vi "Scan DQMH Modules and create Maps.vi"(6 "TreeControl in":refnum<vi>, 7 "Data Cluster In":T2, 8 "error in":errorcluster, 11 "Scan DQMH Modules Argument":T1) -> (0 "error out":errorcluster, 5 "Data Cluster Out":T2={"Maps"={"Tree Map"={}}, "DQMH Scan Results"={"All DQMH Modules Refs"=[], "All Modules Descriptions"=[], "All Modules type"=[], "Project References"={"Project Ref"=refnum, "Project Name"="", "Target"=refnum, "App Ref"=refnum}, "Dependencies"=[]}, "Current Selection"={"VI Ref"=refnum, "DQMH Lib Ref"=refnum}, "Module type"=enum."Singleton", "Module ID"=-1, "Theme"=FALSE, "Broadcast?"=FALSE, "Root Path"="", "Tree Selection"=""})   [LabVIEW 2019, in "Panther Dashboard.lvlib"]
doc: "Gets the Singleton and Cloneable references and creates a list of each type of DQMH Modules"
uses:
  Panther Dashboard.lvlib
  Module Data--cluster.ctl
  Maps List and refs--cluster.ctl
  <vilib>/National Instruments/Tree Map/Tree Map Data.ctl
  DQMH Modules Info--cluster.ctl
  Module type--enum.ctl
  Project References--cluster.ctl
  Scan DQMH Modules Argument--cluster.ctl
  <vilib>/National Instruments/Tree Map/API/List Roots.vi
  <vilib>/National Instruments/Tree Map/Utility/Into Tree Control Items.vi
  <vilib>/Delacor/Delacor QMH/Libraries/Scripting API/DQMH_Scripting API.lvlib
  <vilib>/National Instruments/Tree Map/Tree Map.lvlib
panel:
  out "Pretty XML":string
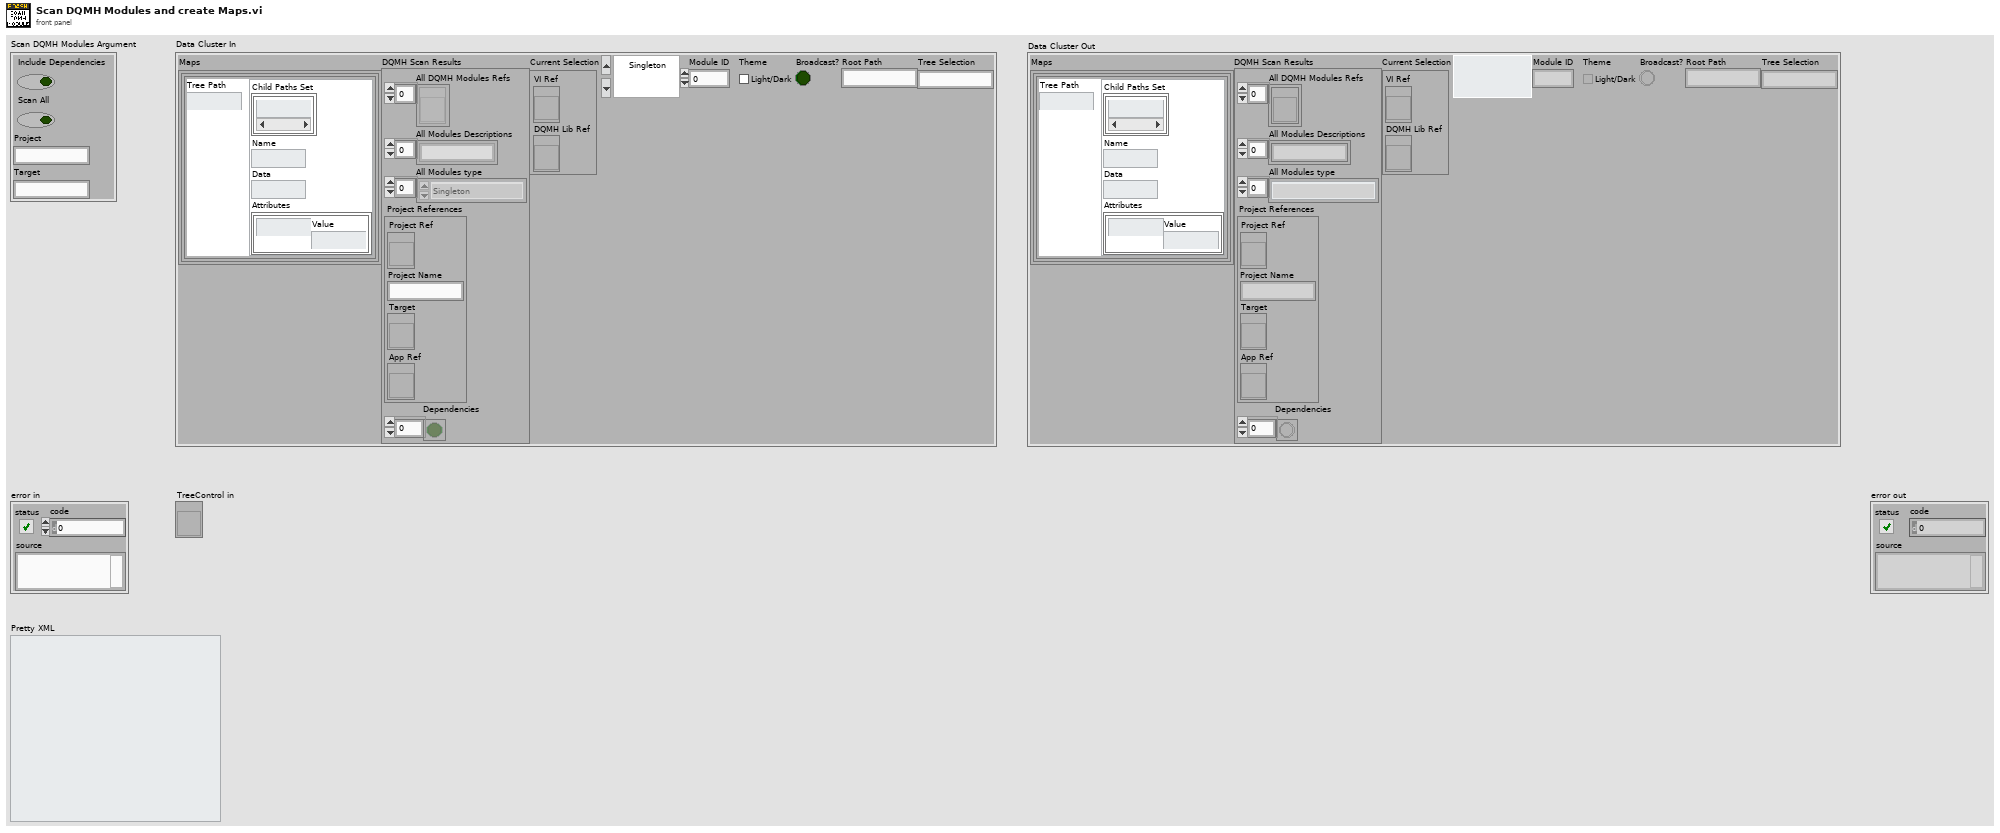
[diagram p1: front panel]
types:
  T1 = typedef "Panther Dashboard.lvlib/Scan DQMH Modules Argument--cluster.ctl" = cluster{"Include Dependencies":bool, "Scan All":bool, "Project":string, "Target":string}
  T2 = typedef "Panther Dashboard.lvlib/Module Data--cluster.ctl" = cluster{"Maps":T3, "DQMH Scan Results":T5, "Current Selection":cluster{"VI Ref":refnum<vi>, "DQMH Lib Ref":refnum<vi>}, "Module type":T6, "Module ID":i32, "Theme":bool, "Broadcast?":bool, "Root Path":string, "Tree Selection":string}
  T3 = typedef "Panther Dashboard.lvlib/Maps List and refs--cluster.ctl" = cluster{"Tree Map":T4}
  T4 = typedef "Tree Map.lvlib/Tree Map Data.ctl" = map{string, cluster{"Child Paths Set":set{string}, "Name":string, "Data":string, "Attributes":map{string, string}}}
  T5 = typedef "Panther Dashboard.lvlib/DQMH Modules Info--cluster.ctl" = cluster{"All DQMH Modules Refs":refnum<vi>[], "All Modules Descriptions":string[], "All Modules type":T6[], "Project References":T7, "Dependencies":bool[]}
  T6 = typedef "Panther Dashboard.lvlib/Module type--enum.ctl" = enum16{"Singleton", "Cloneable"}
  T7 = typedef "Panther Dashboard.lvlib/Project References--cluster.ctl" = cluster{"Project Ref":refnum<vi>, "Project Name":string, "Target":refnum<vi>, "App Ref":refnum<vi>}
  T8 = typedef "DQMH_Scripting API.lvlib/Module Information--cluster.ctl" = cluster{"Library":refnum<vi>, "Qualified Name":string, "Path":path, "Cloneable":bool, "Under Dependencies":bool}
  T9 = cluster{"Left Cell String":string, "Child Text":string[], "Child Tag":string, "Item Indent":i32, "Child Only?":bool, "Glyph Index":i32}[]
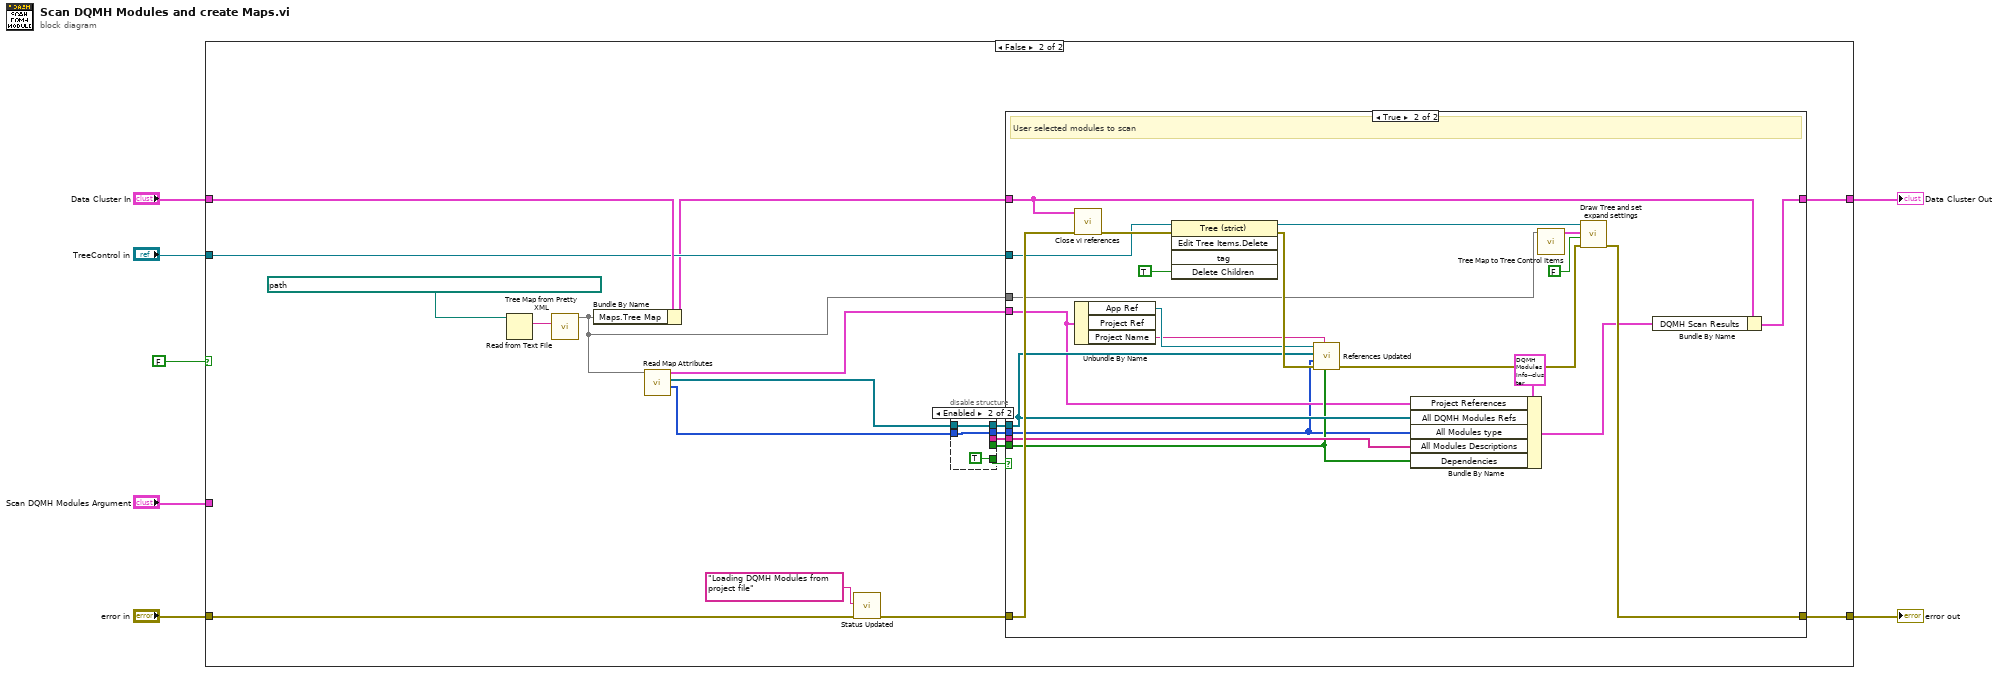
[diagram p0: block diagram]
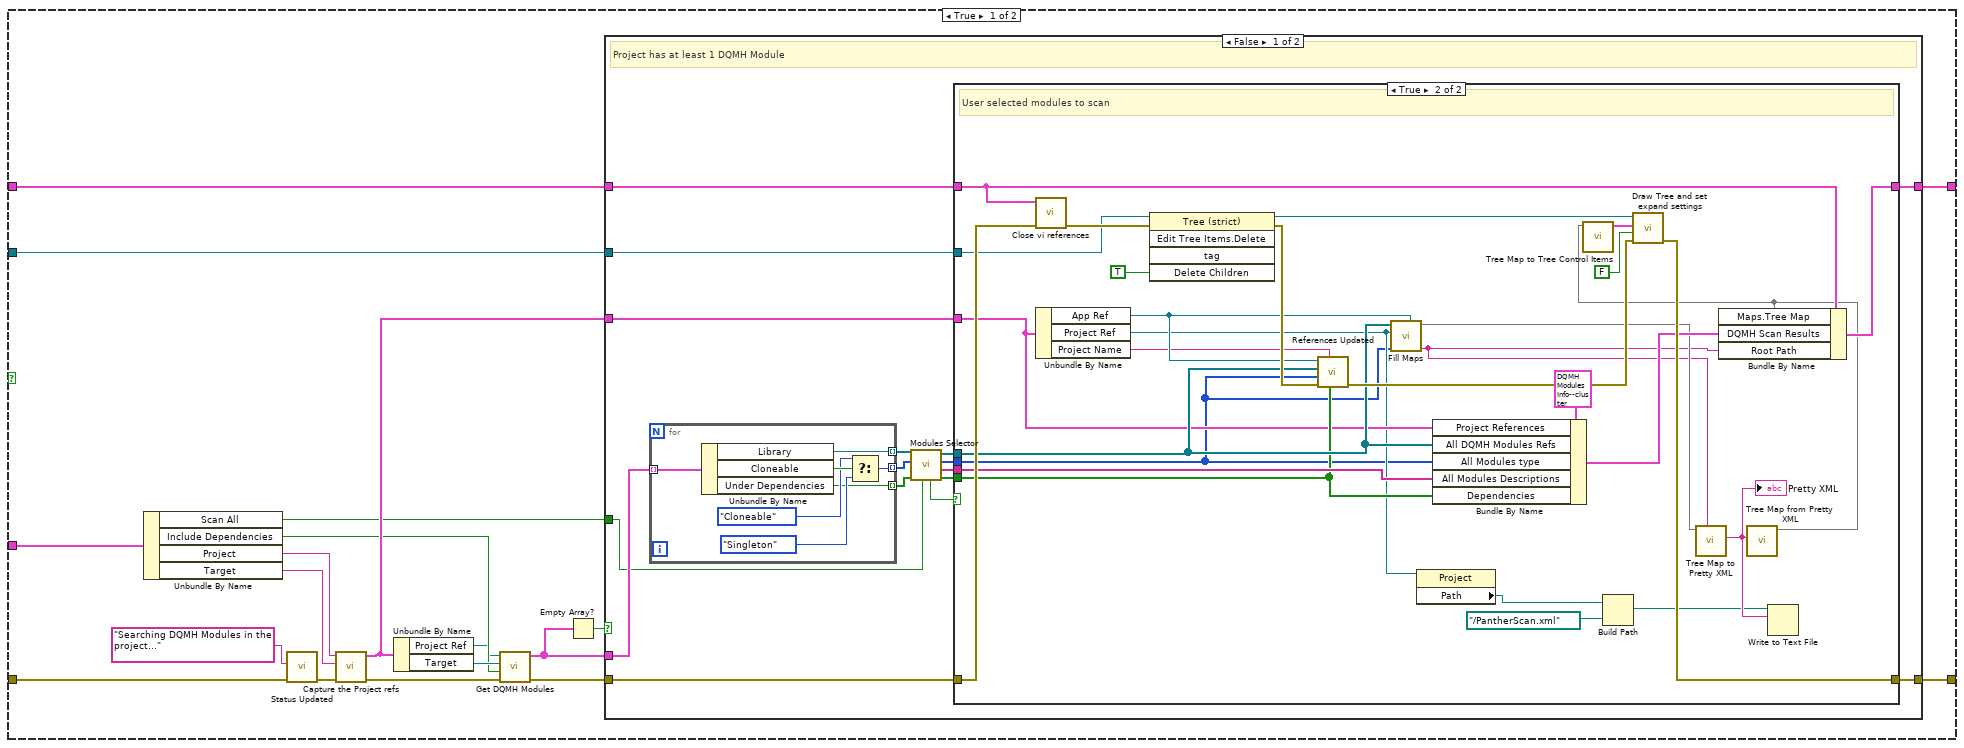
[diagram p2: hidden frame]
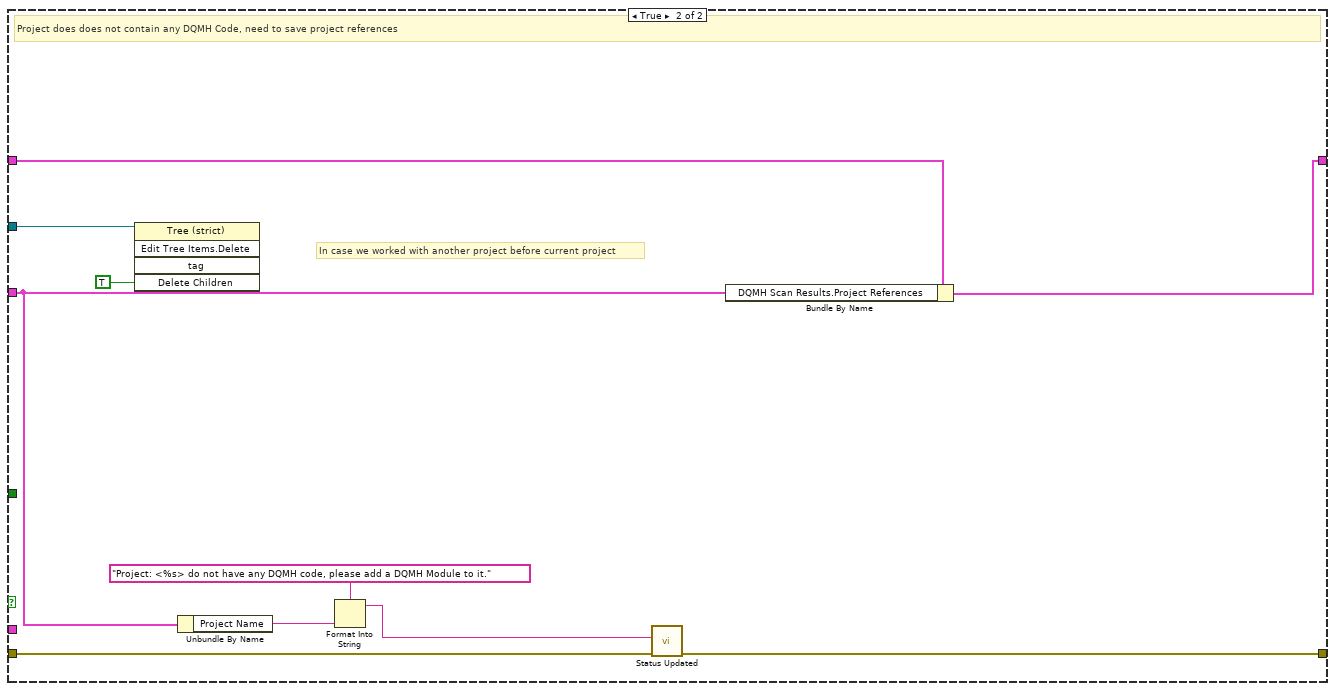
[diagram p4: hidden frame]
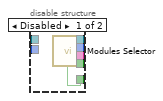
[diagram p5: hidden frame]
diagram:
  n1 = case shown="False" FALSE {
    tunnel: "error in" -> [w25 w108]
    tunnel: [w22 w107] -> w6
    tunnel: "Data Cluster In" -> [w18 w105]
    tunnel: [w17 w104] -> w4
    tunnel: "TreeControl in" -> [w16 w103]
    tunnel: "Scan DQMH Modules Argument" -> [w13 _]
    frame True {
      n2 = Unbundle By Name(w13) -> ("Scan All"=w11:bool, "Include Dependencies"=w12:bool, "Project"=w9:string, "Target"=w10:string)
      n3 = call "Status Updated.vi"("error in (no error)"=w25, "Status"="Searching DQMH Modules in the project...") -> ("error out"=w24:errorcluster)  [unwired: 9 in]
      n4 = call "Capture the Project refs.vi"("error in"=w24, "Target Selection"=w10, "Project Selection"=w9) -> ("error out"=w26:errorcluster, "References"=w19:T7)  [unwired: 7 in]
      n5 = Unbundle By Name(w19) -> ("Project Ref"=w8:refnum<vi>, "Target"=w20:refnum<vi>)
      n6 = call <vilib>:"Get DQMH Modules.vi"("error in"=w26, "Include Dependencies (F)"=w12, "Target (My Computer)"=w20, "Project"=w8) -> ("error out"=w23:errorcluster, "DQMH Modules"=w14:T8[])  [unwired: 6 in]
      n7 = Empty Array?(array=w14) -> (empty?=w15:bool)
      n8 = case shown="False" w15 {
        tunnel: w23 -> [w42 w90]
        tunnel: [w41 w89] -> w22
        tunnel: w19 -> [w37 w86]
        tunnel: w18 -> [w35 w88]
        tunnel: [w34 w87] -> w17
        tunnel: w16 -> [w32 w81]
        tunnel: w14 -> [w31 _]
        tunnel: w11 -> [w27 _]
        frame False {
          # "Project has at least 1 DQMH Module"
          n9 = for {
            tunnel: w31 -> [w80] mode=indexing
            tunnel: [w79] -> w30 mode=indexing
            tunnel: [w75] -> w29 mode=indexing
            tunnel: [w74] -> w28 mode=indexing
            n10 = Unbundle By Name(w80) -> ("Library"=w79:refnum<vi>, "Cloneable"=w77:bool, "Under Dependencies"=w74:bool)
            n11 = Select(t=Module_type--enum."Cloneable", s=w77, f=Module_type--enum."Singleton" ("Module type")) -> (s? t:f=w75:T6)
          }
          n12 = call "Modules Selector.vi"("Scan All"=w27, "Module In Dependencies?"=w28, "Modules Types In"=w29, "DQMH Modules In"=w30) -> ("Module In Dependencies?Out"=w36:bool[], "Descriptions"=w40:string[], "Modules Types Out"=w39:T6[], "DQMH Modules Out"=w38:refnum<vi>[], "Scan?"=w33:bool)  [unwired: 3 in]
          n13 = case shown="True" w33 {
            tunnel: w40 -> [_ w67]
            tunnel: w39 -> [_ w45]
            tunnel: w38 -> [_ w65]
            tunnel: w37 -> [_ w55]
            tunnel: w36 -> [_ w64]
            tunnel: w35 -> [w43 w61]
            tunnel: [w43 w62] -> w34
            tunnel: w32 -> [_ w59]
            tunnel: w42 -> [w44 w71]
            tunnel: [w44 w69] -> w41
            frame False {
              # "User Cancel Scan process, do not redraw tree and keep previous selection"
            }
            frame True {
              # "User selected modules to scan"
              n14 = call "Close vi references.vi"("error in"=w71, "Data Cluster"=w61) -> ("error out"=w73:errorcluster)  [unwired: 9 in]
              n15 = Unbundle By Name(w55) -> ("App Ref"=w66:refnum<vi>, "Project Ref"=w46:refnum<vi>, "Project Name"=w47:string)
              n16 = invoke class="Tree (strict)" method="Edit Tree Items.Delete"(reference=w59, error in=w73, "Delete Children"=TRUE ("Delete Children?")) -> (reference out=w57:refnum<vi>, error out=w72:errorcluster)  [unwired: 2 in, 3 out]
              n17 = call "References Updated.vi"("Dependencies"=w64, "Project Name"=w47, "error in"=w72, "Modules Types"=w45, "Modules"=w65, "Application Instance"=w66) -> ("error out"=w70:errorcluster)  [unwired: 5 in]
              n18 = call "Fill Maps.vi"("App Ref"=w66, "Modules Types"=w45, "Project Ref"=w46, "DQMH Modules"=w65) -> ("Root Path"=w52:string, "Tree Map out"=w54:T4)  [unwired: 6 in]
              n19 = property class="Project"(reference=w46) -> ("Path"=w51:path)  [unwired: 1 in, 2 out]
              n20 = Bundle By Name(cluster=T5 {"All DQMH Modules Refs"=[], "All Modules Descriptions"=[], "All Modules type"=[], "Project References"={"Project Ref"=refnum, "Project Name"="", "Target"=refnum, "App Ref"=refnum}, "Dependencies"=[]} ("DQMH Scan Results"), "Project References"=w55, "All DQMH Modules Refs"=w65, "All Modules type"=w45, "All Modules Descriptions"=w67, "Dependencies"=w64) -> (w63:T5)
              n21 = Build Path(base path=w51, name or relative path=path "../PantherScan.xml") -> (appended path=w48:path)
              n22 = call <vilib>:"Tree Map to Pretty XML.vi"("Root Path"=w52, "Tree Map In"=w54) -> ("Pretty XML"=w49:string)  [unwired: 8 in, 1 out]
              "Pretty XML" <- w49
              n23 = call <vilib>:"Tree Map from Pretty XML.vi"("Pretty XML"=w49) -> ("Tree Map Out"=w53:T4)  [unwired: 9 in, 1 out]
              n24 = call <vilib>:"Tree Map to Tree Control Items.vi"("Tree Map In"=w53) -> ("Tree Control Items"=w60:T9)  [unwired: 10 in]
              n25 = call "Draw Tree and set expand settings.vi"("error in"=w70, "Expanded Results?"=FALSE, "Tree Control Items"=w60, "TreeControl in"=w57) -> ("error out"=w69:errorcluster)  [unwired: 7 in]
              n26 = Bundle By Name(cluster=w61, "Maps.Tree Map"=w53, "DQMH Scan Results"=w63, "Root Path"=w52) -> (w62:T2)
              n27 = Write to Text File(file (use dialog)=w48, text=w49) -> ()  [unwired: 2 in, 3 out]
            }
          }
        }
        frame True {
          # "In case we worked with another project before current project"
          # "Project does does not contain any DQMH Code, need to save project references"
          n28 = invoke class="Tree (strict)" method="Edit Tree Items.Delete"(reference=w81, "Delete Children"=TRUE ("Delete Children?")) -> ()  [unwired: 3 in, 5 out]
          n29 = Unbundle By Name(w86) -> ("Project Name"=w85:string)
          n30 = Format Into String(format string="Project: <%s> do not have any DQMH code, please add a DQMH Module to it.", w85) -> (resulting string=w84:string)  [unwired: 2 in, 1 out]
          n31 = call "Status Updated.vi"("error in (no error)"=w90, "Status"=w84) -> ("error out"=w89:errorcluster)  [unwired: 9 in]
          n32 = Bundle By Name(cluster=w88, "DQMH Scan Results.Project References"=w86) -> (w87:T2)
        }
      }
    }
    frame False {
      n33 = Read from Text File(file (use dialog)=path "C:/Users/Enrique Noé Arias/Desktop/Untitled Project 1/PantherScan.xml") -> (text=w96:string)  [unwired: 3 in, 3 out]
      n34 = call <vilib>:"Tree Map from Pretty XML.vi"("Pretty XML"=w96) -> ("Tree Map Out"=w91:T4)  [unwired: 9 in, 1 out]
      n35 = Bundle By Name(cluster=w105, "Maps.Tree Map"=w91) -> (w95:T2)
      n36 = call "Read Map Attributes.vi"("Tree Map In (empty)"=w91) -> ("Modules Types Out"=w92:T6[], "Library References"=w93:refnum<vi>[], "References"=w94:T7)  [unwired: 7 in, 1 out]
      n37 = call "Status Updated.vi"("error in (no error)"=w108, "Status"="Loading DQMH Modules from project file") -> ("error out"=w109:errorcluster)  [unwired: 9 in]
      n38 = disable-structure shown="Enabled" {
        disable-tunnel: [w114 _] -> w102
        disable-tunnel: [w113 w116] -> w101
        disable-tunnel: [w112 w117] -> w100
        disable-tunnel: [w111 _] -> w99
        disable-tunnel: [w110 TRUE ("Scan?")] -> w98
        disable-tunnel: w93 -> [_ w117]
        disable-tunnel: w92 -> [_ w116]
        frame Disabled {
          n39 = call "Modules Selector.vi"() -> ("Module In Dependencies?Out"=w111:bool[], "Descriptions"=w114:string[], "Modules Types Out"=w113:T6[], "DQMH Modules Out"=w112:refnum<vi>[], "Scan?"=w110:bool)  [unwired: 7 in]
        }
        frame Enabled {
        }
      }
      n40 = case shown="True" w98 {
        tunnel: w102 -> [_ w135]
        tunnel: w101 -> [_ w121]
        tunnel: w100 -> [_ w133]
        tunnel: w94 -> [_ w123]
        tunnel: w99 -> [_ w132]
        tunnel: w95 -> [w118 w129]
        tunnel: [w118 w130] -> w104
        tunnel: w103 -> [_ w127]
        tunnel: w109 -> [w119 w139]
        tunnel: [w119 w137] -> w107
        tunnel: w91 -> [_ w120]
        frame False {
          # "User Cancel Scan process, do not redraw tree and keep previous selection"
        }
        frame True {
          # "User selected modules to scan"
          n41 = call "Close vi references.vi"("error in"=w139, "Data Cluster"=w129) -> ("error out"=w141:errorcluster)  [unwired: 9 in]
          n42 = Unbundle By Name(w123) -> ("App Ref"=w134:refnum<vi>, "Project Name"=w122:string)  [unwired: 1 out]
          n43 = invoke class="Tree (strict)" method="Edit Tree Items.Delete"(reference=w127, error in=w141, "Delete Children"=TRUE ("Delete Children?")) -> (reference out=w125:refnum<vi>, error out=w140:errorcluster)  [unwired: 2 in, 3 out]
          n44 = call "References Updated.vi"("Dependencies"=w132, "Project Name"=w122, "error in"=w140, "Modules Types"=w121, "Modules"=w133, "Application Instance"=w134) -> ("error out"=w138:errorcluster)  [unwired: 5 in]
          n45 = Bundle By Name(cluster=T5 {"All DQMH Modules Refs"=[], "All Modules Descriptions"=[], "All Modules type"=[], "Project References"={"Project Ref"=refnum, "Project Name"="", "Target"=refnum, "App Ref"=refnum}, "Dependencies"=[]} ("DQMH Scan Results"), "Project References"=w123, "All DQMH Modules Refs"=w133, "All Modules type"=w121, "All Modules Descriptions"=w135, "Dependencies"=w132) -> (w131:T5)
          n46 = call <vilib>:"Tree Map to Tree Control Items.vi"("Tree Map In"=w120) -> ("Tree Control Items"=w128:T9)  [unwired: 10 in]
          n47 = call "Draw Tree and set expand settings.vi"("error in"=w138, "Expanded Results?"=FALSE, "Tree Control Items"=w128, "TreeControl in"=w125) -> ("error out"=w137:errorcluster)  [unwired: 7 in]
          n48 = Bundle By Name(cluster=w129, "DQMH Scan Results"=w131) -> (w130:T2)
        }
      }
    }
  }
  "error out" <- w6
  "Data Cluster Out" <- w4
